vi "String_Get File Extention from file name.vi"(11 "Path String":string) -> (2 "Filename Without Extension Out":string, 3 "Lowercase File Extension Out":string)   [LabVIEW 2015]
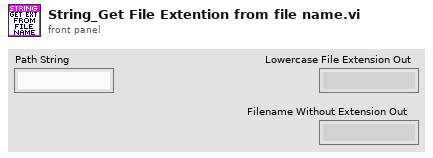
[diagram p1: front panel]
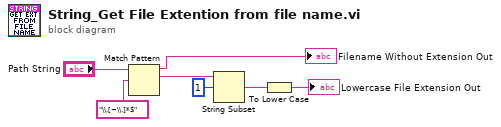
[diagram p0: block diagram]
diagram:
  n1 = Match Pattern(string="Path String", regular expression="\\.[~\\.]*$") -> (before substring=→"Filename Without Extension Out":string, match substring=w4:string)  [unwired: 3 out]
  n2 = String Subset(string=w4, offset (0)=1) -> (substring=w5:string)  [unwired: 1 out]
  n3 = To Lower Case(string=w5) -> (all lower case string=→"Lowercase File Extension Out":string)
